vi "PLC释放.vi"(8 "错误输入（无错误） 2":errorcluster caption="错误输入（无错误）", 11 "引用":refnum<k24>) -> (0 "错误输入（无错误）":errorcluster)   [LabVIEW 2021]
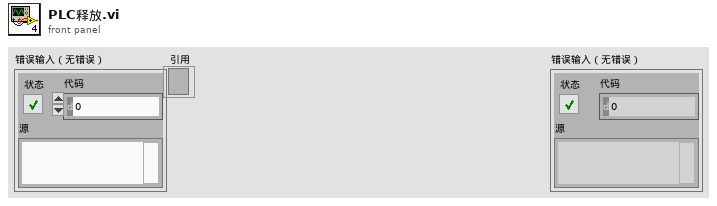
[diagram p1: front panel]
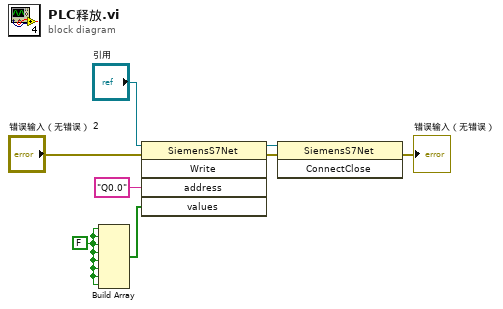
[diagram p0: block diagram]
diagram:
  w1 = FALSE
  n1 = Build Array(w1, w1, w1, w1, w1, w1, w1, w1) -> (w7:bool[])
  n2 = invoke class="SiemensS7Net" method="Write"(reference="引用", error in="错误输入（无错误） 2", "address"="Q0.0", "values"=w7) -> (reference out=w6:refnum<k24>, error out=w5:errorcluster)  [unwired: 1 in, 3 out]
  n3 = invoke class="SiemensS7Net" method="ConnectClose"(reference=w6, error in=w5) -> (error out=→"错误输入（无错误）":errorcluster)  [unwired: 1 in, 2 out]
